vi "MRC Ds Comms Control Set Op Mode Options.vi"(8 "error in (no error)":errorcluster, 11 "opModes":T1[](array[typedef])) -> (0 "error out":errorcluster)   [LabVIEW 2026, in "MrcLib.lvlib"]
doc: "MRC_Status MRC_CALLCONV MRC_DsCommsControl_SetOpModeOptions(struct MRC_OpMode* opModes, uint16_t opModeCount);"
uses:
  MrcLib.lvlib
  Types/MRC OpMode.ctl
  Types/MRC Name 64.ctl
  MrcLib.dll
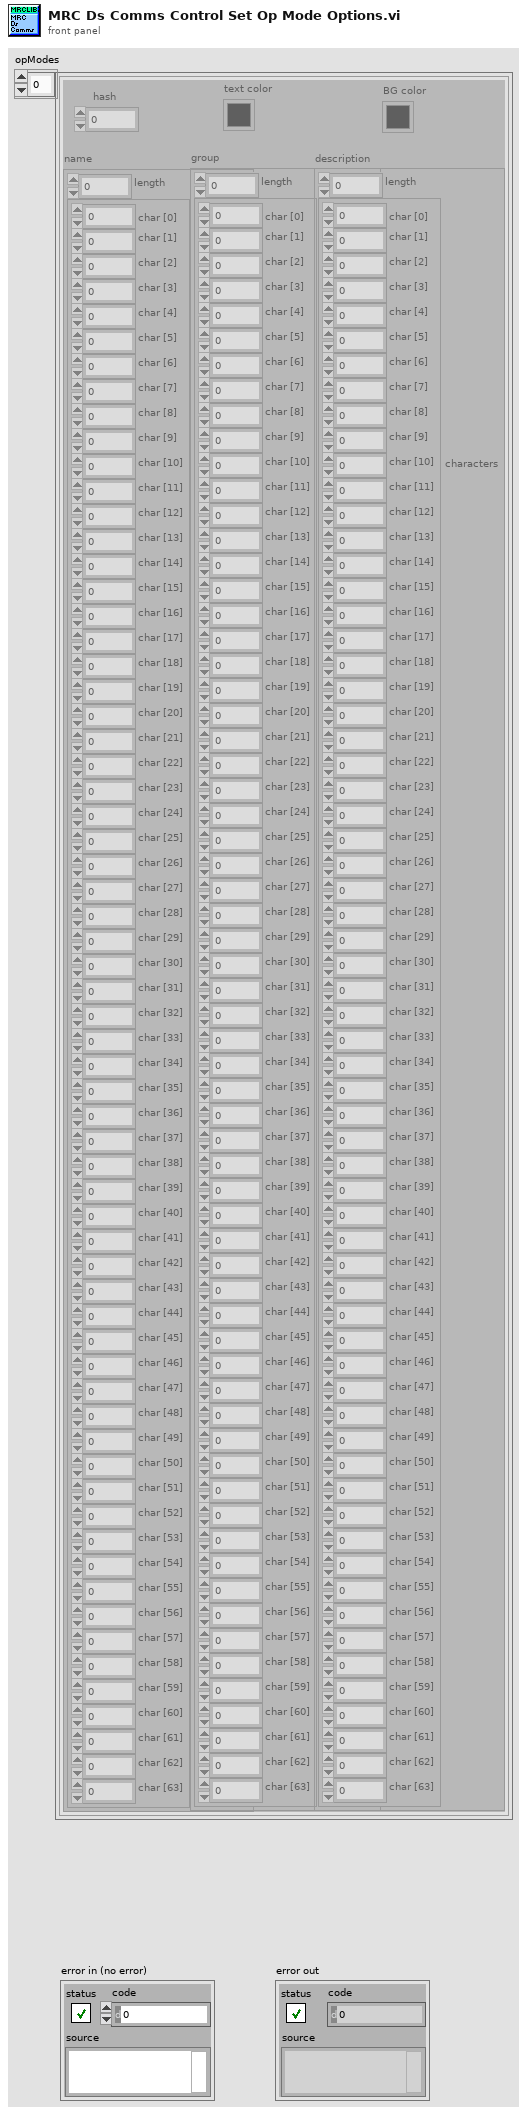
[diagram p1: front panel]
types:
  T1 = typedef "MRC OpMode.ctl" = cluster{"hash":u64, "name":T2, "group":T2, "description":T2, "text color":u32, "BG color":u32}
  T2 = typedef "MRC Name 64.ctl" = cluster{"length":u8, "characters":cluster{"char [63]":i8, "char [62]":i8, "char [61]":i8, "char [60]":i8, "char [59]":i8, "char [58]":i8, "char [57]":i8, "char [56]":i8, "char [55]":i8, "char [54]":i8, "char [53]":i8, "char [52]":i8, "char [51]":i8, "char [50]":i8, "char [49]":i8, "char [48]":i8, "char [47]":i8, "char [46]":i8, "char [45]":i8, "char [44]":i8, "char [43]":i8, "char [42]":i8, "char [41]":i8, "char [40]":i8, "char [39]":i8, "char [38]":i8, "char [37]":i8, "char [36]":i8, "char [35]":i8, "char [34]":i8, "char [33]":i8, "char [32]":i8, "char [31]":i8, "char [30]":i8, "char [29]":i8, "char [28]":i8, "char [27]":i8, "char [26]":i8, "char [25]":i8, "char [24]":i8, "char [23]":i8, "char [22]":i8, "char [21]":i8, "char [20]":i8, "char [19]":i8, "char [18]":i8, "char [17]":i8, "char [16]":i8, "char [15]":i8, "char [14]":i8, "char [13]":i8, "char [12]":i8, "char [11]":i8, "char [10]":i8, "char [9]":i8, "char [8]":i8, "char [7]":i8, "char [6]":i8, "char [5]":i8, "char [4]":i8, "char [3]":i8, "char [2]":i8, "char [1]":i8, "char [0]":i8}}
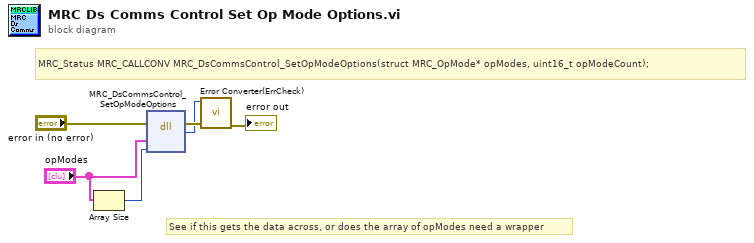
[diagram p0: block diagram]
diagram:
  # "See if this gets the data across, or does the array of opModes need a wrapper"
  # "MRC_Status MRC_CALLCONV MRC_DsCommsControl_SetOpModeOptions(struct MRC_OpMode* opModes, uint16_t opModeCount);"
  n1 = Array Size(array="opModes") -> (size(s)=w1:i32)
  n2 = dll-call lib="MrcLib.*" fn="MRC_DsCommsControl_SetOpModeOptions"(error in="error in (no error)", "opModes"="opModes", "opModeCount"=w1) -> (error out=w5:errorcluster, "return type"=w3:i32)  [unwired: 4 in, 1 out]
  n3 = call "Error Converter(ErrCheck).vi"("error in (no error)"=w5, "status"=w3) -> ("error out"=→"error out":errorcluster)  [unwired: 9 in]
